vi "InsertIntoSubpanel.vi"(8 "error in (no error)":errorcluster, 10 "VI Ref":refnum<vi>, 11 "Subpanel":refnum<vi>) -> (0 "error out":errorcluster)   [LabVIEW 2019, in "UserInterface.lvlib"]
uses:
  UserInterface.lvlib
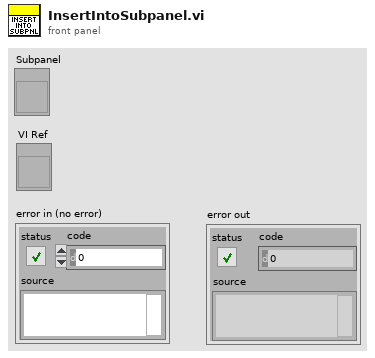
[diagram p1: front panel]
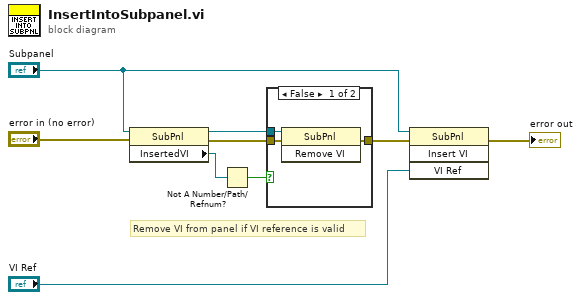
[diagram p0: block diagram]
diagram:
  # "Remove VI from panel if VI reference is valid"
  n1 = property class="SubPnl"(reference="Subpanel", error in="error in (no error)") -> (reference out=w5:refnum<vi>, error out=w6:errorcluster, "InsertedVI"=w4:refnum<vi>)
  n2 = Not A Number/Path/Refnum?(number/path/refnum=w4) -> (NaN/Path/Refnum?=w3:bool)
  n3 = case shown="False" w3 {
    tunnel: [w12 w13] -> w8
    tunnel: w6 -> [w11 w13]
    tunnel: w5 -> [w10 _]
    frame False {
      n4 = invoke class="SubPnl" method="Remove VI"(reference=w10, error in=w11) -> (error out=w12:errorcluster)  [unwired: 1 in, 2 out]
    }
    frame True {
    }
  }
  n5 = invoke class="SubPnl" method="Insert VI"(reference="Subpanel", error in=w8, "VI Ref"="VI Ref") -> (error out=→"error out":errorcluster)  [unwired: 1 in, 3 out]
